vi "FTW-Actor-ShutdownEventLogger.vi"(0 "FTW Actor":refnum<class "FTW-Actor.lvclass">, 11 "error in":errorcluster) -> (4 "FTW Actor out":refnum<class "FTW-Actor.lvclass">, 15 "error out":errorcluster)   [LabVIEW 2014, in "FTW-Actor.lvclass"]
uses:
  FTW-Actor.lvclass
  Logging/FTW-EventLogger-API.lvclass
panel:
  # "Inputs"
  # "Outputs"
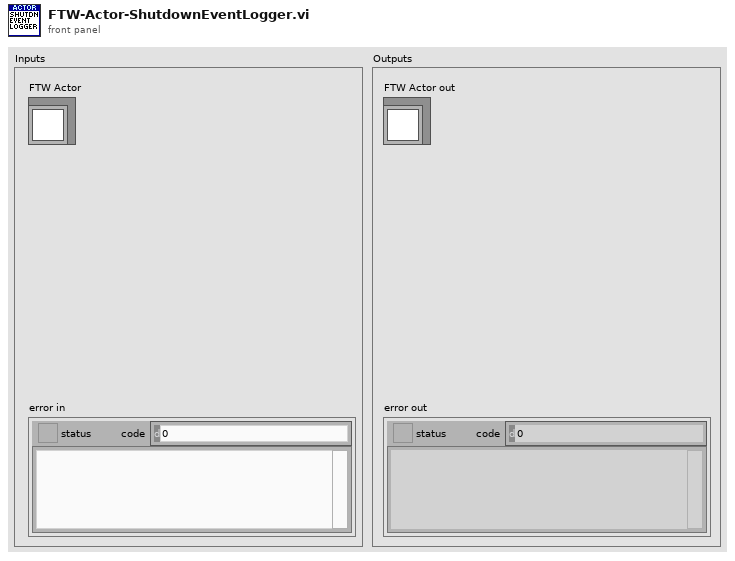
[diagram p1: front panel]
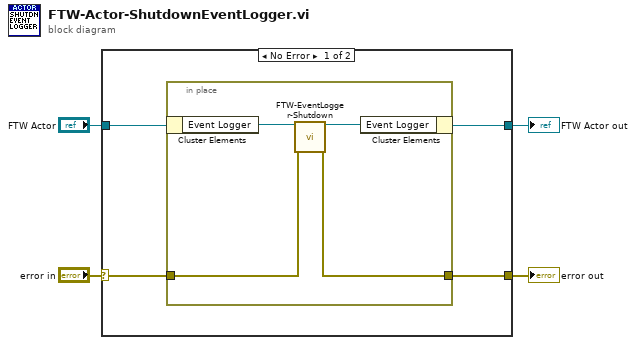
[diagram p0: block diagram]
diagram:
  n1 = case shown="No Error" "error in" {
    selector: "error in" -> [w8 w13]
    tunnel: [w6 w13] -> w4
    tunnel: "FTW Actor" -> [w7 w14]
    tunnel: [w5 w14] -> w2
    frame No Error {
      n2 = in-place {
        in-place-border: w8 -> [w12]
        in-place-border: [w9] -> w6
        n3 = in-place-cluster #1(w7) -> ("Event Logger"=w11:refnum<class "FTW-EventLogger-API.lvclass">)
        n4 = call "FTW-EventLogger-Shutdown.vi"("Event Logger API"=w11, "error in"=w12) -> ("Event Logger API out"=w10:refnum<class "FTW-EventLogger-API.lvclass">, "error out"=w9:errorcluster)  [unwired: 12 in]
        n5 = in-place-cluster #1("Event Logger"=w10) -> (w5:refnum<class "FTW-Actor.lvclass">)
      }
    }
    frame Error {
    }
  }
  "error out" <- w4
  "FTW Actor out" <- w2
